vi "MS_architecture.vi"() -> ()   [LabVIEW 2020]
panel:
  in  "stop":bool
  in  "Speak":bool
  out "Slave 2":string
  out "Slave 1":string
  out "error out":errorcluster
  in  "error in (no error)":errorcluster
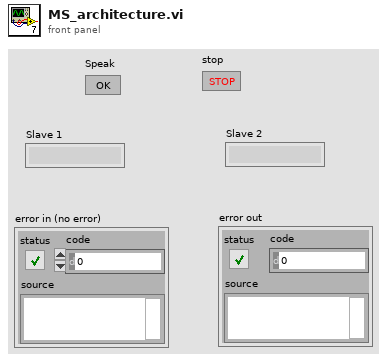
[diagram p1: front panel]
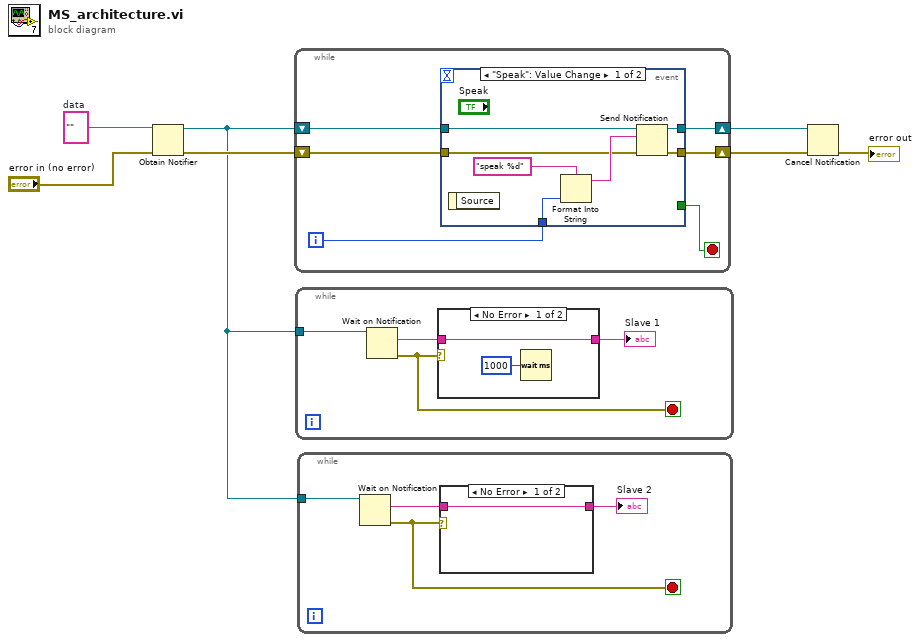
[diagram p0: block diagram]
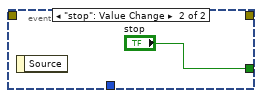
[diagram p4: hidden frame]
diagram:
  w2 = ""  # data
  n1 = Obtain Notifier(notification data type=w2, error in (no error)="error in (no error)") -> (notifier out=w3:refnum<notifier>, error out=w6:errorcluster)  [unwired: 2 in, 1 out]
  n2 = while {
    shift-right: [w10] -> w4
    shift-left: w3 -> [w9]
    shift-right: [w8] -> w1
    shift-left: w6 -> [w11]
    i -> [w13]
    stop <- w12 stop-if-true
    n3 = event shown="[0] \"Speak\": Value Change" {
      selector: _ -> [_ _]
      dyn-events: _ -> [_ _]
      timeout: _ -> [_ _]
      tunnel: w13 -> [w20 _]
      tunnel: w11 -> [w16 _]
      tunnel: [_ "stop"] -> w12
      tunnel: w9 -> [w17 _]
      tunnel: [w15 _] -> w10
      tunnel: [w14 _] -> w8
      event "Speak": Value Change {
        n4 = event-data() -> ()  [unwired: 1 in, 1 out]
        n5 = Format Into String(format string="speak %d", w20) -> (resulting string=w18:string)  [unwired: 2 in, 1 out]
        n6 = Send Notification(notification=w18, notifier=w17, error in (no error)=w16) -> (notifier out=w15:refnum<notifier>, error out=w14:errorcluster)
      }
      event "stop": Value Change {
        n7 = event-data() -> ()  [unwired: 1 in, 1 out]
      }
    }
  }
  n8 = while {
    tunnel: w3 -> [w25]
    stop <- w22 stop-if-true
    n9 = Wait on Notification(notifier=w25) -> (notification=w24:string, error out=w22:errorcluster)  [unwired: 3 in, 2 out]
    n10 = case shown="No Error" w22 {
      tunnel: w24 -> [w27 w28]
      tunnel: [w27 w28] -> w23
      frame No Error {
        n11 = Wait (ms)(milliseconds to wait=u32 1000) -> ()  [unwired: 1 out]
      }
      frame Error {
      }
    }
    "Slave 1" <- w23
  }
  n12 = while {
    tunnel: w3 -> [w32]
    stop <- w31 stop-if-true
    n13 = Wait on Notification(notifier=w32) -> (notification=w30:string, error out=w31:errorcluster)  [unwired: 3 in, 2 out]
    n14 = case shown="No Error" w31 {
      tunnel: w30 -> [w33 w34]
      tunnel: [w33 w34] -> w29
      frame No Error {
      }
      frame Error {
      }
    }
    "Slave 2" <- w29
  }
  n15 = Cancel Notification(0:w4, 3:w1) -> (11:→"error out":errorcluster)  [unwired: 2 out]
